vi "Write Text to Screen.vi"(8 "error in (no error)":errorcluster, 9 "text":string, 11 "VISA session":refnum<visa-resource-name>) -> (0 "error out":errorcluster, 3 "dup VISA session":refnum<visa-resource-name>)   [LabVIEW 2018, in "Agilent 87XX Series.lvlib"]
doc: "This VI for the HP8753 Network Analyzer is used to write text to the screen. Unlike the regular title feature as implemented in the \"display title\" VI, text generated with this VI can be longer than 50 characters. As is each line should be no more than 70 characters and the total number of lines should be less than or equal to 34. Exceeding these limits can cause \"screen garbage\" as nothing is done in the VI to check these limits.\n\n New lines should be delineated by a line feed. \n\n The GPIB address used by this VI should be the primary address of the Network Analyzer and not the address of the CRT.\n\n The text can be cleared by writing blank text to the instrument.\n\n Text written with the \"write text to screen\" VI is always plotted even if everything is turned off (except the plotter of course). It is plotted in the color of the text pen."
uses:
  Agilent 87XX Series.lvlib
panel:
  in  "VISA session (for class)":refnum<visa-resource-name>
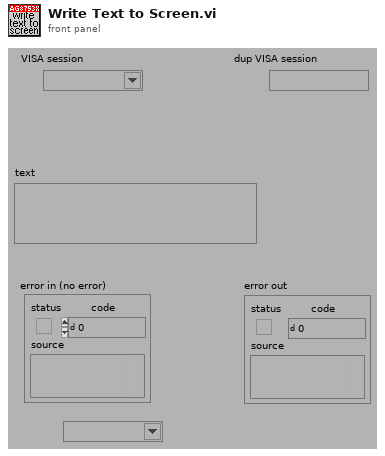
[diagram p1: front panel]
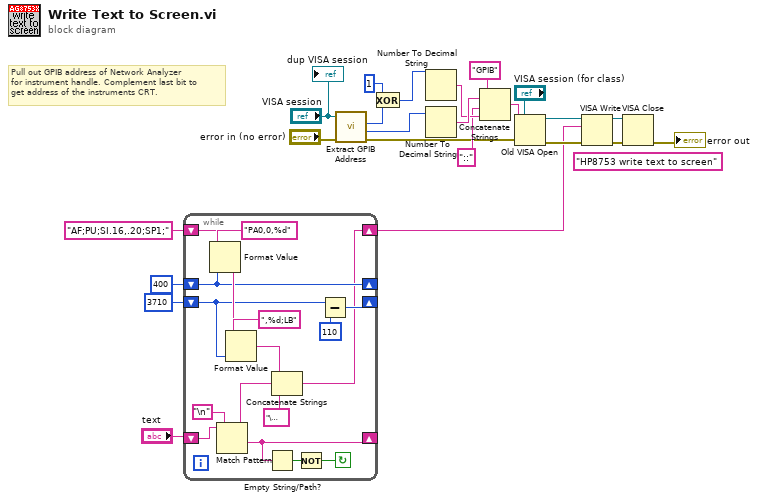
[diagram p0: block diagram]
diagram:
  (unwired) "HP8753 write text to screen"
  # "Pull out GPIB address of Network Analyzer\nfor instrument handle. Complement last bit to\nget address of the instruments CRT."
  n1 = while {
    shift-left: "AF;PU;SI.16,.20;SP1;" -> [w25]
    shift-right: [w24] -> w5
    shift-left: "text" -> [w33]
    shift-right: [w29] -> _
    shift-left: 3710 -> [w26]
    shift-right: [w35] -> _
    shift-left: 400 -> [w37]
    shift-right: [w37] -> _
    stop <- w27 continue-if-true
    n2 = Format Value(string ("")=w25, format string="PA0,0,%d", value (0)=w37) -> (output string=w38:string)
    n3 = Match Pattern(string=w33, regular expression="\n") -> (before substring=w31:string, after substring=w29:string)  [unwired: 1 in, 2 out]
    n4 = Format Value(string ("")=w38, format string=",%d;LB", value (0)=w26) -> (output string=w32:string)
    n5 = Empty String/Path?(string/path=w29) -> (empty?=w28:bool)
    n6 = Concatenate Strings(w32, w31, "\u0003;") -> (w24:string)
    n7 = Not(x=w28) -> (.not. x?=w27:bool)
    n8 = Subtract(x=w26, y=110) -> (x-y=w35:i32)
  }
  n9 = call "Extract GPIB Address.VI"("error in (no error)"="error in (no error)", "VISA resource name"="VISA session") -> ("error out"=w4:errorcluster, "GPIB Board"=w2:u16, "GPIB address"=w18:u16)  [unwired: 6 in, 1 out]
  n10 = Exclusive Or(1:w18, 2:1) -> (0:w3:i32)
  n11 = Number To Decimal String(number=w3) -> (decimal integer string=w7:string)  [unwired: 1 in]
  n12 = Number To Decimal String(number=w2) -> (decimal integer string=w8:string)  [unwired: 1 in]
  n13 = Concatenate Strings("GPIB", w8, "::", w7) -> (w10:string)
  n14 = Old VISA Open(8:w4, 10:w10, 11:"VISA session (for class)") -> (0:w12:errorcluster, 3:w11:refnum<visa-resource-name>)  [unwired: 2 in]
  n15 = VISA Write(VISA resource name=w11, write buffer=w5, error in (no error)=w12) -> (VISA resource name out=w14:refnum<visa-resource-name>, error out=w15:errorcluster)  [unwired: 1 out]
  n16 = VISA Close(VISA resource name=w14, error in (no error)=w15) -> (error out=→"error out":errorcluster)
  "dup VISA session" <- "VISA session"
